vi "Read Log with Size Limit.vi"(7 "size limit":i64=131072, 8 "error in (no error)":errorcluster, 11 "Info Log":path) -> (0 "error out":errorcluster, 3 "Log":string)   [LabVIEW 2021, in "CIFPluginManager.lvclass"]
uses:
  CIFPluginManager.lvclass
  CIFPluginManager.lvclass/CIFPluginManager.ctl
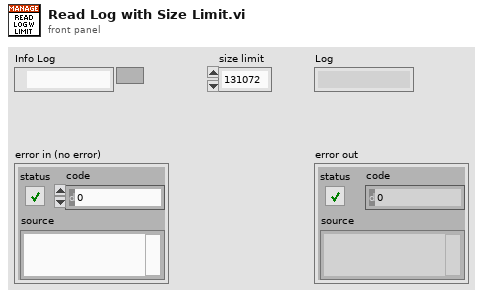
[diagram p1: front panel]
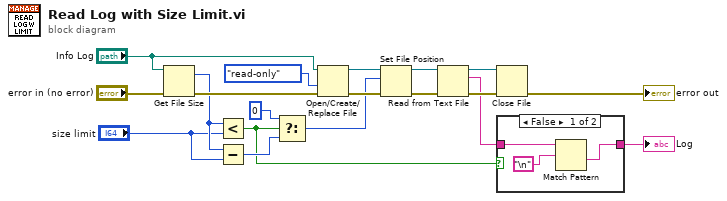
[diagram p0: block diagram]
diagram:
  n1 = Get File Size(file="Info Log", error in="error in (no error)") -> (size (in bytes)=w12:i64, 0:w13:errorcluster)  [unwired: 1 out]
  n2 = Less?(x=w12, y="size limit") -> (x < y?=w2:bool)
  n3 = Subtract(x=w12, y="size limit") -> (x-y=w6:i64)
  n4 = Select(t=i64 0, s=w2, f=w6) -> (s? t:f=w4:i64)
  n5 = Open/Create/Replace File(file path (use dialog)="Info Log", error in=w13, access (0:read/write)=enum16{"read/write", "read-only", "write-only"}."read-only") -> (refnum out=w9:refnum<file>, error out=w10:errorcluster)  [unwired: 3 in, 1 out]
  n6 = Set File Position(offset (in bytes) (0)=w4, refnum=w9, error in=w10) -> (refnum out=w7:refnum<file>, error out=w8:errorcluster)  [unwired: 1 in]
  n7 = Read from Text File(file (use dialog)=w7, error in=w8) -> (refnum out=w16:refnum<file>, text=w3:string, error out=w17:errorcluster)  [unwired: 2 in, 1 out]
  n8 = Close File(refnum=w16, error in=w17) -> (error out=→"error out":errorcluster)  [unwired: 1 out]
  n9 = case shown="False" w2 {
    tunnel: w3 -> [w21 w23]
    tunnel: [w20 w23] -> w1
    frame False {
      n10 = Match Pattern(string=w21, regular expression="\n") -> (after substring=w20:string)  [unwired: 1 in, 3 out]
    }
    frame True {
    }
  }
  "Log" <- w1
